vi "J1939 Data Lookup Table.vi"(6 "command":T3, 7 "Direct Access":cluster{"Offset":u32, "Length":u32}, 8 "error in (no error)":errorcluster {"code" min=0 max=0}, 9 "Signals":dbl[](array[numeric]), 10 "ID":u32, 11 "scaling information":T1) -> (0 "error out":errorcluster {"code" min=0 max=0}, 1 "Signals Out":dbl[](array[numeric]))   [LabVIEW 2013, in "J1939.lvlib"]
uses:
  J1939.lvlib
  J1939 Data Lookup Table Action.ctl
  API Types/Scaling Initialization.ctl
  CD/CD Conversion Lookup Table Parameters Cluster.ctl
  Frame Conversion/Common Conversions.vi
  Frame Conversion/Convert CAN Arb ID to J1939 ID.vi
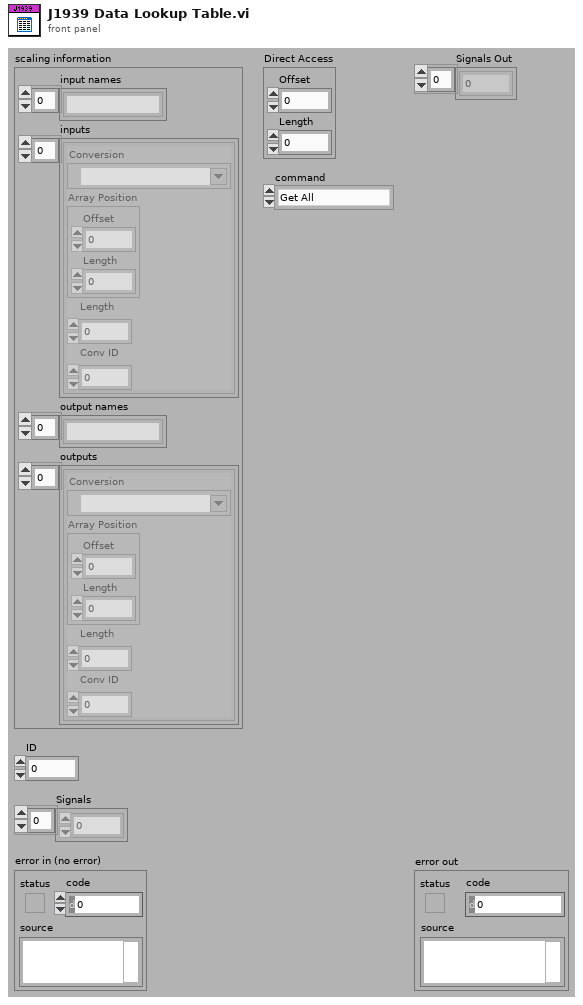
[diagram p1: front panel]
types:
  T1 = typedef "J1939.lvlib/scaling initialization.ctl" = cluster{"input names":string[], "inputs":T2[], "output names":string[], "outputs":T2[]}
  T2 = typedef "J1939.lvlib/CD Conversion Lookup Table Parameters Cluster.ctl" = cluster{"Conversion":refnum<k21>, "Array Position":cluster{"Offset":u32, "Length":u32}, "Length":u32, "Conv ID":u32}
  T3 = typedef "J1939.lvlib/J1939 Data Lookup Table Action.ctl" = enum16{"Get All", "Set All", "Set Frame", "Get Frame", "Set Range", "Get Range"}
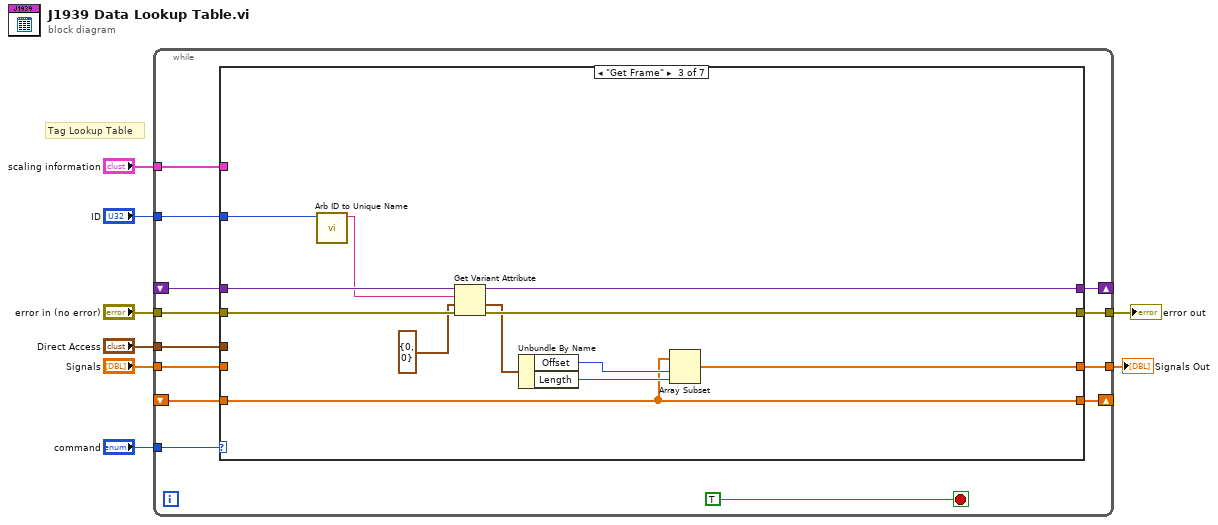
[diagram p0: block diagram]
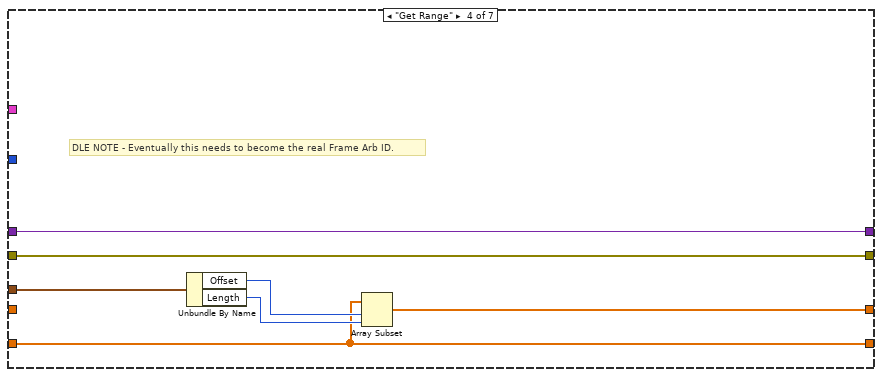
[diagram p4: hidden frame]
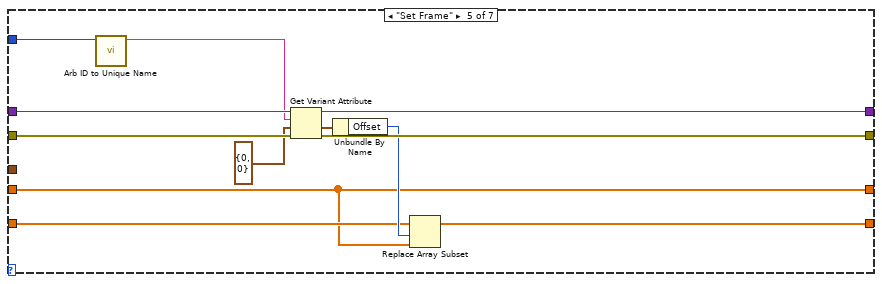
[diagram p5: hidden frame]
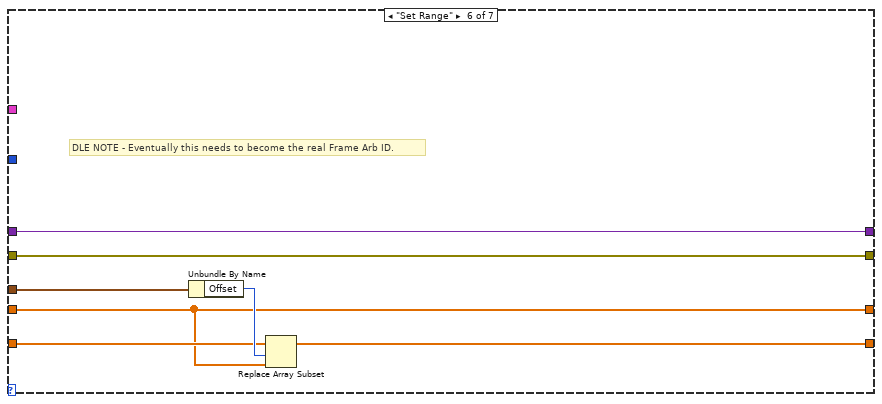
[diagram p6: hidden frame]
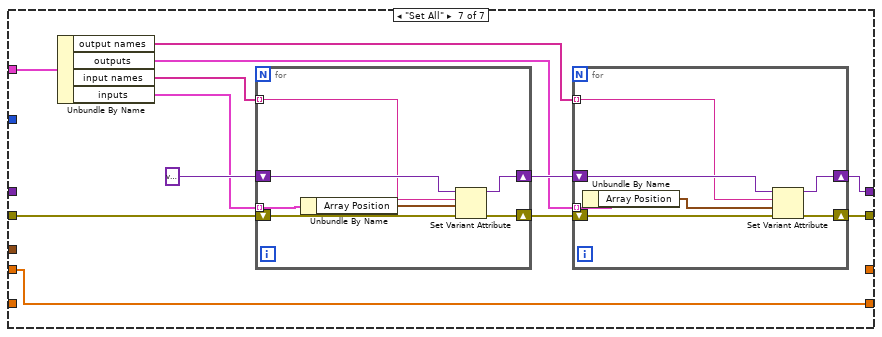
[diagram p7: hidden frame]
diagram:
  # "Tag Lookup Table"
  n1 = while {
    shift-right: [w10] -> _
    shift-left: _ -> [w19]
    tunnel: "command" -> [w20]
    tunnel: "error in (no error)" -> [w18]
    tunnel: [w17] -> w6
    tunnel: "ID" -> [w16]
    shift-right: [w15] -> _
    shift-left: _ -> [w14]
    tunnel: [w13] -> w3
    tunnel: "Signals" -> [w12]
    tunnel: "Direct Access" -> [w11]
    tunnel: "scaling information" -> [w9]
    stop <- TRUE stop-if-true
    n2 = case shown="\"Get Frame\"" w20 {
      tunnel: w19 -> [w23 w25 w37 w39 w56 w58 _]
      tunnel: w18 -> [_ _ w36 w40 w55 w57 w74]
      tunnel: [_ _ w34 w40 w53 w57 w68] -> w17
      tunnel: w16 -> [_ _ w27 _ w46 _ _]
      tunnel: [w22 w24 w28 w41 w48 w61 w65] -> w15
      tunnel: w14 -> [w22 w24 w28 w41 w49 w62 _]
      tunnel: [_ w24 w29 w42 w47 w60 _] -> w13
      tunnel: w12 -> [_ _ _ _ w47 w60 w65]
      tunnel: w11 -> [_ _ _ w38 _ w59 _]
      tunnel: [w23 w25 w35 w39 w54 w58 w69] -> w10
      tunnel: w9 -> [_ _ _ _ _ _ w64]
      frame Default {
      }
      frame "Get All" {
      }
      frame "Get Frame" {
        n3 = call "Arb ID to Unique Name.vi"("Arb ID"=w27) -> ("name"=w26:string)  [unwired: 10 in]
        n4 = Get Variant Attribute(Variant=w37, name=w26, default value (empty Variant)=cluster{"Offset":u32, "Length":u32} {"Offset"=0, "Length"=0} ("Channel Array Position"), error in=w36) -> (duplicate Variant=w35:variant, value=w32:cluster{"Offset":u32, "Length":u32}, error out=w34:errorcluster)  [unwired: 1 out]
        n5 = Unbundle By Name(w32) -> ("Offset"=w30:u32, "Length"=w31:u32)
        n6 = Array Subset(array=w28, index=w30, length=w31) -> (w29:dbl[])
      }
      frame "Get Range" {
        # "DLE NOTE - Eventually this needs to become the real Frame Arb ID."
        n7 = Unbundle By Name(w38) -> ("Offset"=w43:u32, "Length"=w44:u32)
        n8 = Array Subset(array=w41, index=w43, length=w44) -> (w42:dbl[])
      }
      frame "Set Frame" {
        n9 = call "Arb ID to Unique Name.vi"("Arb ID"=w46) -> ("name"=w45:string)  [unwired: 10 in]
        n10 = Get Variant Attribute(Variant=w56, name=w45, default value (empty Variant)=cluster{"Offset":u32, "Length":u32} {"Offset"=0, "Length"=0} ("Channel Array Position"), error in=w55) -> (duplicate Variant=w54:variant, value=w51:cluster{"Offset":u32, "Length":u32}, error out=w53:errorcluster)  [unwired: 1 out]
        n11 = Unbundle By Name(w51) -> ("Offset"=w50:u32)
        n12 = Replace Array Subset(array=w49, new element=w47, index=w50) -> (w48:dbl[])
      }
      frame "Set Range" {
        # "DLE NOTE - Eventually this needs to become the real Frame Arb ID."
        n13 = Unbundle By Name(w59) -> ("Offset"=w63:u32)
        n14 = Replace Array Subset(array=w62, new element=w60, index=w63) -> (w61:dbl[])
      }
      frame "Set All" {
        n15 = Unbundle By Name(w64) -> ("output names"=w67:string[], "outputs"=w66:T2[], "input names"=w73:string[], "inputs"=w72:T2[])
        n16 = for {
          shift-right: [w88] -> w70
          shift-left: variant ("variant") -> [w89]
          shift-right: [w86] -> w71
          shift-left: w74 -> [w87]
          tunnel: w73 -> [w85] mode=indexing
          tunnel: w72 -> [w84] mode=indexing
          n17 = Unbundle By Name(w84) -> ("Array Position"=w83:cluster{"Offset":u32, "Length":u32})
          n18 = Set Variant Attribute(Variant=w89, name=w85, value=w83, error in=w87) -> (Variant out=w88:variant, error out=w86:errorcluster)  [unwired: 1 out]
        }
        n19 = for {
          shift-right: [w81] -> w69
          shift-left: w70 -> [w82]
          shift-right: [w79] -> w68
          shift-left: w71 -> [w80]
          tunnel: w67 -> [w78] mode=indexing
          tunnel: w66 -> [w77] mode=indexing
          n20 = Unbundle By Name(w77) -> ("Array Position"=w76:cluster{"Offset":u32, "Length":u32})
          n21 = Set Variant Attribute(Variant=w82, name=w78, value=w76, error in=w80) -> (Variant out=w81:variant, error out=w79:errorcluster)  [unwired: 1 out]
        }
      }
    }
  }
  "error out" <- w6
  "Signals Out" <- w3
